vi "Write Local Optimization Iterations.vi"(8 "error in (no error)":errorcluster, 10 "Local Optimization Iterations":i32=5, 11 "USAC Params in":refnum<class "USAC Params.lvclass">) -> (0 "error out":errorcluster, 3 "USAC Params out":refnum<class "USAC Params.lvclass">)   [LabVIEW 2020, in "ar.lvlib" / "USAC Params.lvclass"]
doc: "Write Local Optimization Iterations.\n\nSee https://docs.opencv.org/4.10.0/de/d3e/tutorial_usac.html for more information on usage and note that not all combinations of parameters will be valid."
uses:
  USAC Params.lvclass
  USAC Params.lvclass/USAC Params.ctl
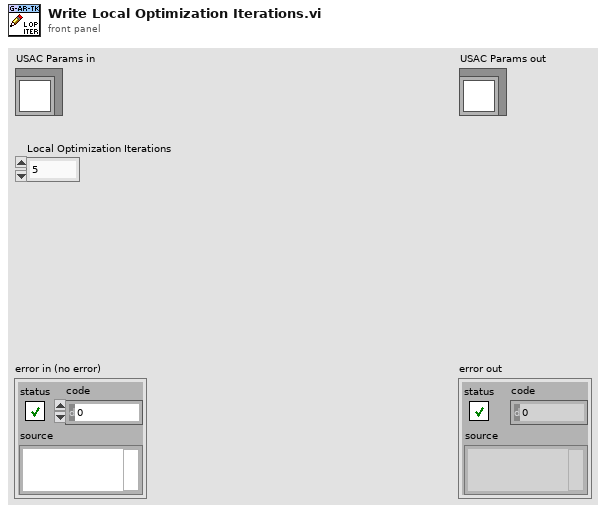
[diagram p1: front panel]
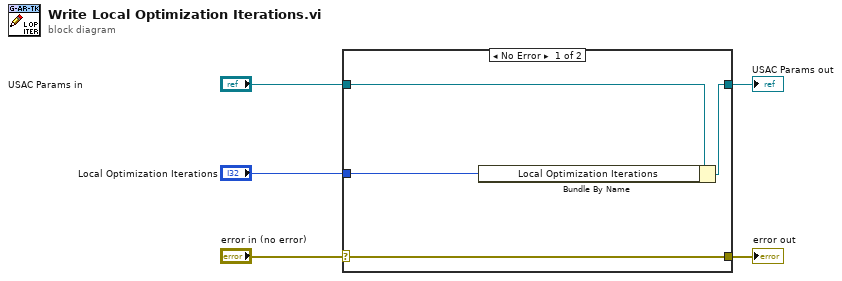
[diagram p0: block diagram]
diagram:
  n1 = case shown="No Error" "error in (no error)" {
    selector: "error in (no error)" -> [w9 w10]
    tunnel: [w9 w10] -> w4
    tunnel: [w7 w11] -> w2
    tunnel: "USAC Params in" -> [w8 w11]
    tunnel: "Local Optimization Iterations" -> [w6 _]
    frame No Error {
      n2 = Bundle By Name(cluster=w8, "Local Optimization Iterations"=w6) -> (w7:refnum<class "USAC Params.lvclass">)
    }
    frame Error {
    }
  }
  "error out" <- w4
  "USAC Params out" <- w2
